vi "OnResume.vi"(8 "error in (no error)":errorcluster, 11 "Pong in":refnum<class "Pong.lvclass">) -> (0 "error out":errorcluster, 3 "Pong out":refnum<class "Pong.lvclass">)   [LabVIEW 2019]
uses:
  Pong.lvclass
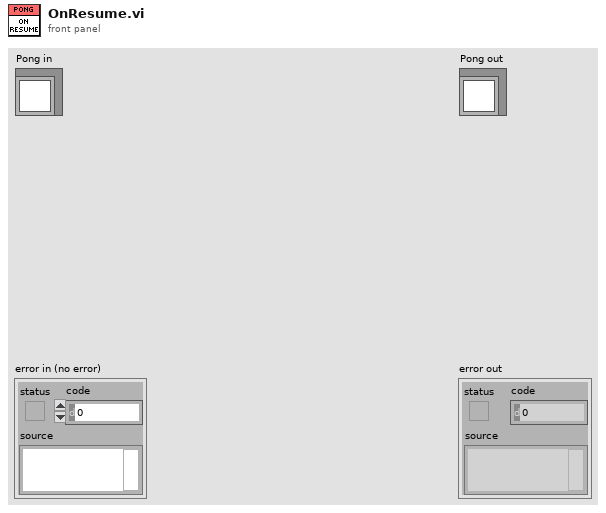
[diagram p1: front panel]
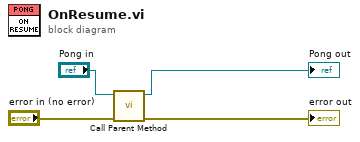
[diagram p0: block diagram]
diagram:
  n1 = call-parent "Call Parent Method"("error in (no error)"="error in (no error)", "Game in"="Pong in") -> ("error out"=→"error out":errorcluster, "Game out"=→"Pong out":refnum<class "Pong.lvclass">)  [unwired: 8 in]
